vi "Analysis.DeterminePass.vi"(8 "error in (no error)":errorcluster, 11 "Properties":variant) -> (0 "error out":errorcluster, 2 "Passed?":bool)   [LabVIEW 2015, in "Analysis.lvlib"]
uses:
  Analysis.lvlib
  Types/Analysis.PropertyGroups.ctl
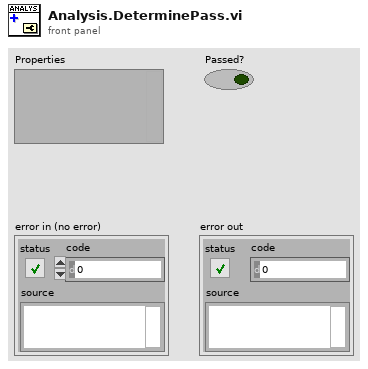
[diagram p1: front panel]
types:
  T1 = typedef "Analysis.lvlib/Analysis.PropertyGroups.ctl" = cluster{"Pass":bool, "Additional Info":variant}
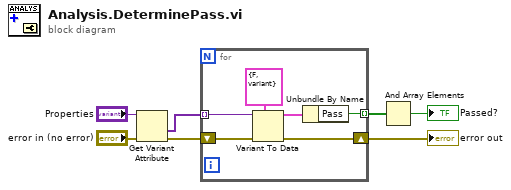
[diagram p0: block diagram]
diagram:
  n1 = Get Variant Attribute(Variant="Properties", error in="error in (no error)") -> (values=w6:variant[], error out=w5:errorcluster)  [unwired: 2 in, 2 out]
  n2 = for {
    shift-right: [w8] -> w1
    shift-left: w5 -> [w10]
    tunnel: [w9] -> w2 mode=indexing
    tunnel: w6 -> [w12] mode=indexing
    n3 = Variant To Data(error in=w10, type=T1 {"Pass"=FALSE, "Additional Info"=variant}, Variant=w12) -> (data=w11:T1, error out=w8:errorcluster)
    n4 = Unbundle By Name(w11) -> ("Pass"=w9:bool)
  }
  "error out" <- w1
  n5 = And Array Elements(Boolean array=w2) -> (logical AND=→"Passed?":bool)
